vi "Get Waveform DVRs.vi"(8 "error in (no error)":errorcluster, 9 "Ignore Read Lock":bool, 10 "Number of Waveforms":i32=-2, 11 "DVR Circular Buffer in":refnum<data-value>[](array[refnum])) -> (0 "error out":errorcluster, 1 "Timeout":bool, 2 "DVRs":refnum<data-value>[](array[refnum]), 3 "DVR Circular Buffer out":refnum<data-value>[](array[refnum]))   [LabVIEW 2021, in "ChannelCommon.lvlib"]
uses:
  ChannelCommon.lvlib
  typedef/Datatype Waveform.ctl
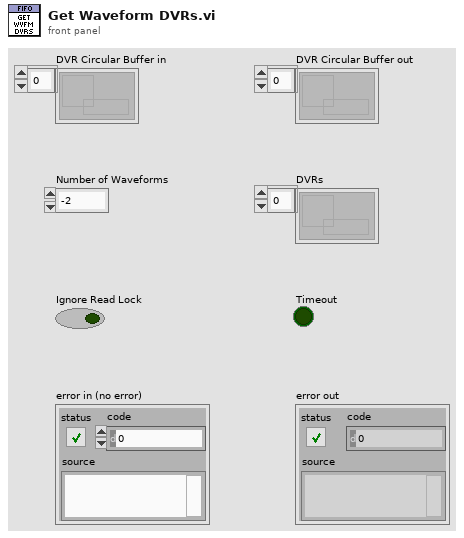
[diagram p1: front panel]
types:
  T1 = typedef "ChannelCommon.lvlib/Datatype Waveform.ctl" = cluster{"measurement":dbl[], "dT":dbl, "Timestamp":u64, "Read Lock":bool}
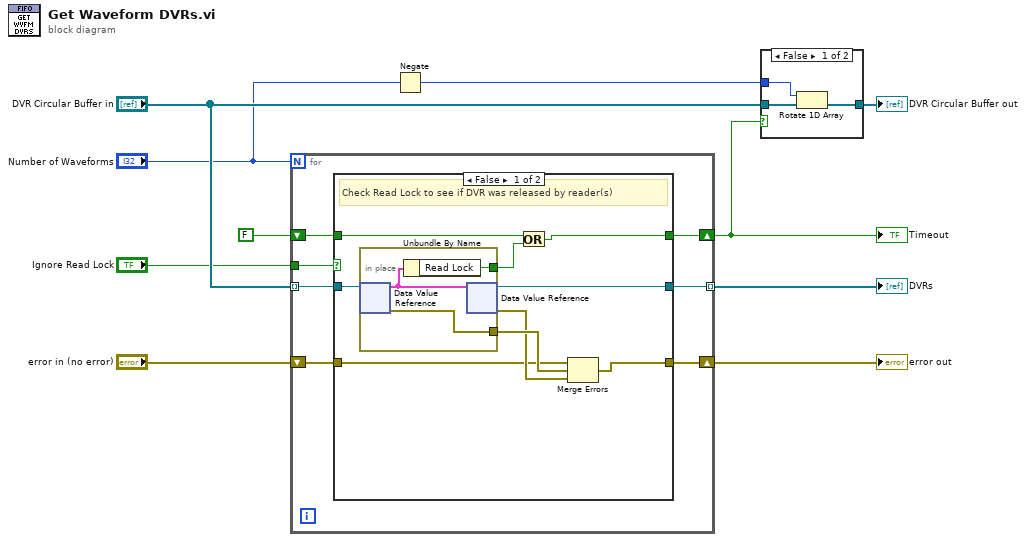
[diagram p0: block diagram]
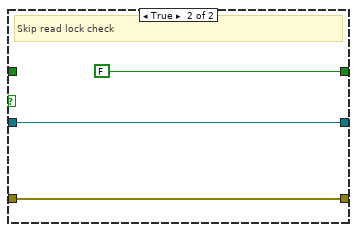
[diagram p2: hidden frame]
diagram:
  n1 = for {
    N: "Number of Waveforms" -> [_]
    tunnel: "DVR Circular Buffer in" -> [w17] mode=indexing
    shift-right: [w13] -> w1
    shift-left: FALSE ("Read Lock") -> [w14]
    tunnel: "Ignore Read Lock" -> [w16]
    tunnel: [w15] -> w7 mode=indexing
    shift-right: [w11] -> w2
    shift-left: "error in (no error)" -> [w12]
    n2 = case shown="False" w16 {
      tunnel: w17 -> [w26 w31]
      tunnel: [w23 w31] -> w15
      tunnel: w14 -> [w22 _]
      tunnel: [w20 FALSE ("Read Lock")] -> w13
      tunnel: w12 -> [w19 w30]
      tunnel: [w18 w30] -> w11
      frame False {
        # "Check Read Lock to see if DVR was released by reader(s)"
        n3 = in-place {
          in-place-border: [w29] -> w21
          in-place-border: [w27] -> w25
          n4 = in-place-dvr #1(w26) -> (w28:T1, w27:errorcluster)
          n5 = Unbundle By Name(w28) -> ("Read Lock"=w29:bool)
          n6 = in-place-dvr #1(w28) -> (w23:refnum<data-value>, w24:errorcluster)
        }
        n7 = Or(x=w22, y=w21) -> (x .or. y?=w20:bool)
        n8 = Merge Errors(w19, w25, w24) -> (w18:errorcluster)
      }
      frame True {
        # "Skip read lock check"
      }
    }
  }
  "Timeout" <- w1
  "error out" <- w2
  "DVRs" <- w7
  n9 = Negate(x="Number of Waveforms") -> (-x=w3:i32)
  n10 = case shown="False" w1 {
    tunnel: "DVR Circular Buffer in" -> [w35 w36]
    tunnel: [w34 w36] -> w10
    tunnel: w3 -> [w33 _]
    frame False {
      n11 = Rotate 1D Array(1:w35, 2:w33) -> (0:w34:refnum<data-value>[])
    }
    frame True {
    }
  }
  "DVR Circular Buffer out" <- w10
